vi "daemon.vi"(8 "error in (no error)":errorcluster, 11 "manager_daemon.lvclass":refnum<class "manager_daemon.lvclass">) -> ()   [LabVIEW 2024, in "manager_daemon.lvclass"]
uses:
  manager_daemon.lvclass
  type_defs/cmd--enum.ctl
  TypeDefs/graphic.filter--cluster.ctl
  Graphic_UI/typedefs/volume.type.colors--cluster.ctl
  manager_daemon.lvclass/manager_daemon.ctl
  CV_Shared_Library/volume.type--enum.ctl
  type_defs/msg--cluster.ctl
  type_defs/PublisherData--cluster.ctl
  type_defs/PublisherMap--map.ctl
  add.sub.to.map.vi
  CV_Shared_Library/open.local.volume.file.vi
  add.publisher.vi
  <userlib>/_OpenG.lib/file/file.llb/Strip Path Extension - String__ogtk.vi
  CV_Shared_Library/open.local.issue.file.vi
  CV_Shared_Library/CV_Shared_Library.lvlib
  <userlib>/_OpenG.lib/file/file.llb/openg_file.lvlib
panel:
  out "iteration":i32
  out "latest filter":T1
  out "Volume changed":path
  out "Issue changed":path
  out "cmd":T3
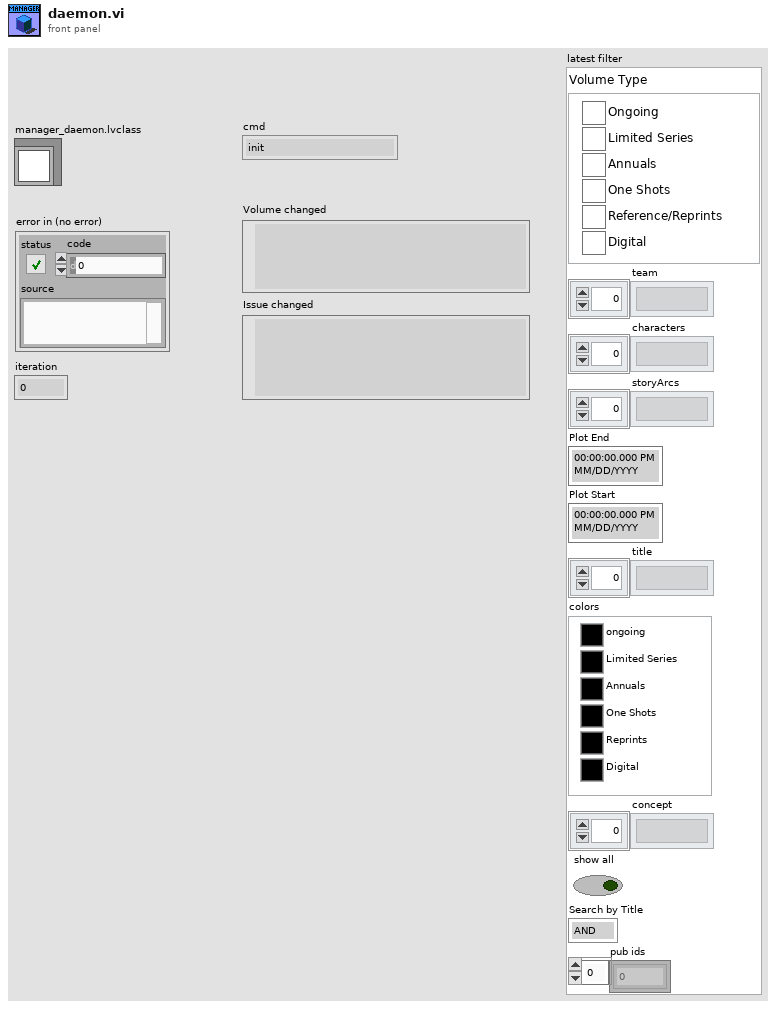
[diagram p1: front panel]
types:
  T1 = typedef "CV_Shared_Library.lvlib/graphic.filter--cluster.ctl" = cluster{"Volume Type":cluster{"Ongoing":bool, "Limited Series":bool, "Annuals":bool, "One Shots":bool, "Reference/Reprints":bool, "Digital":bool}, "team":string[], "characters":string[], "storyArcs":string[], "Plot End":timestamp, "Plot Start":timestamp, "title":string[], "colors":T2, "concept":string[], "show all":bool, "Search by Title":enum32{"AND", "OR"}, "pub ids":i32[]}
  T2 = typedef "volume.type.colors--cluster.ctl" = cluster{"ongoing":u32, "Limited Series":u32, "Annuals":u32, "One Shots":u32, "Reprints":u32, "Digital":u32}
  T3 = typedef "manager_daemon.lvclass/cmd--enum.ctl" = enum16{"init", "run", "load binaries", "save binaries", "updated volume", "get set names", "return vol path by id", "return vol ids by publisher", "display info", "filter release week", "apply filter", "add publisher", "get publishers", "add volume", "save volumes", "add issues", "add issue", "delete volume", "delete issues", "download issues", "scan for reprints", "exit"}
  T4 = cluster{"selection filter":T1, "graph only (f)":bool}
  T5 = cluster{"Volume Path":path, "Update All (T)":bool}
  T6 = typedef "CV_Shared_Library.lvlib/volume.type--enum.ctl" = enum16{"Ongoing", "Limited Series", "Annual", "One Shot", "Reprint/Document", "Digital"}
  T7 = cluster{"search string":string, "source type":T6, "dest type":T6, "publisher":string}
  T8 = typedef "manager_daemon.lvclass/msg--cluster.ctl" = cluster{"cmd":T3, "data":variant}
  T9 = cluster{"Volume Path":i32[], "Update All (T)":bool}
  T10 = cluster{"vol id":i32, "notifier out":refnum<notifier>}
  T11 = cluster{"publisher id":i32, "notifier out":refnum<notifier>}
  T12 = typedef "manager_daemon.lvclass/PublisherData--cluster.ctl" = cluster{"id":i32, "volumes":set{i32}}
  T13 = cluster{"Issue Path":path, "Update All (T)":bool}
  T14 = typedef "manager_daemon.lvclass/sub-map--map.ctl" = map{string, T15}
  T15 = typedef "manager_daemon.lvclass/SubData--cluster.ctl" = cluster{"id":i32, "issues":set{i32}}
  T16 = typedef "manager_daemon.lvclass/binary.references--cluster.ctl" = cluster{"issues.bin ref":refnum<file>, "chars.bin ref":refnum<file>, "concepts.bin ref":refnum<file>, "storys.bin ref":refnum<file>, "teams.bin ref":refnum<file>, "vollumes.bin ref":refnum<file>, "publishers.bin ref":refnum<file>}
  T17 = typedef "manager_daemon.lvclass/VolumeData--cluster.ctl" = cluster{"name":string, "sortable_name":string, "aliases":string[], "description":string, "site_detail_url":string, "count_of_issues":i32, "start_year":i32, "publisher_id":i32, "issue_ids":i32[], "date_last_updated":timestamp, "volume":i32, "cv_id":string, "volume type":T6, "source_path":path}
  T18 = typedef "manager_daemon.lvclass/PublisherMap--map.ctl" = map{string, T12}
  T19 = cluster{"changed volume ids":i32[], "Update All (T)":bool}
  T20 = typedef "CV_RESTful_Lib.lvlib/local_publisher--cluster.ctl" = cluster{"id":i32, "name":string, "sortable_name":string, "aliases":string[], "description":string, "deck":string, "site_detail_url":string, "date_last_updated":timestamp, "cv_id":string, "volume_ids":i32[]}
  T21 = typedef "manager_daemon.lvclass/IssueData--clustrer.ctl" = cluster{"cover_date":timestamp, "cv_id":string, "name":string, "sortable_name":string, "issue_number":string, "deck":string, "description":string, "volume id":i32, "store_date":timestamp, "date_last_updated":timestamp, "site_detail_url":string, "cover_url":string, "source_path":path, "in_collection":bool, "display_date":timestamp}
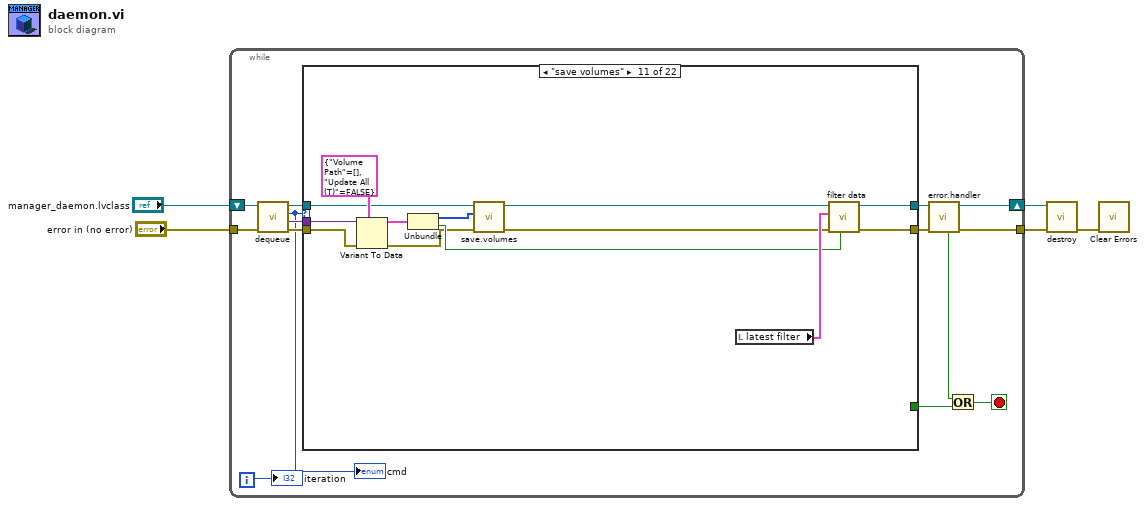
[diagram p0: block diagram]
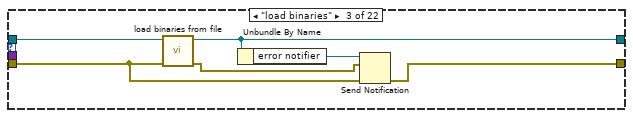
[diagram p4: hidden frame]
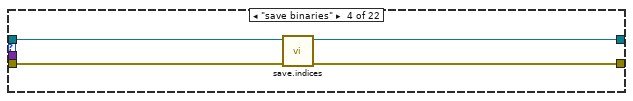
[diagram p5: hidden frame]
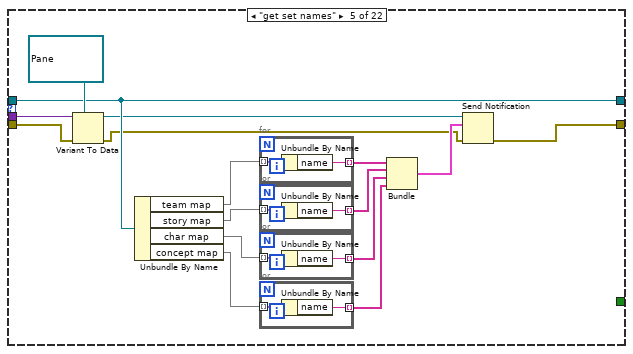
[diagram p6: hidden frame]
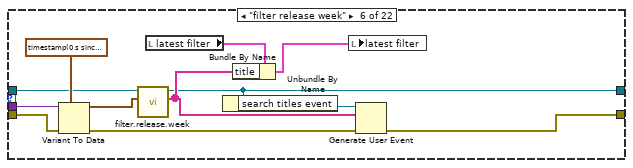
[diagram p7: hidden frame]
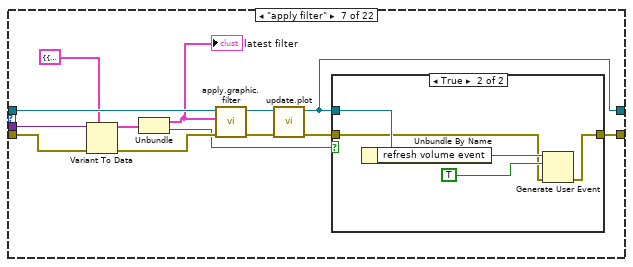
[diagram p8: hidden frame]
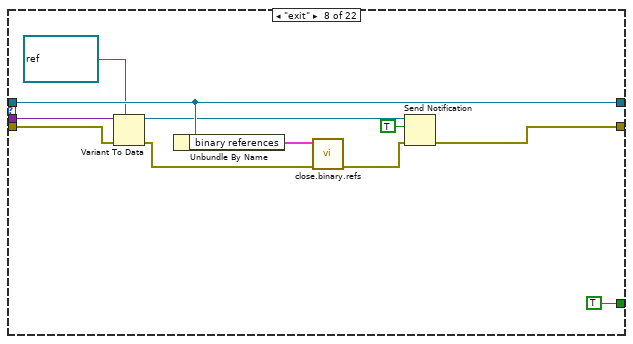
[diagram p10: hidden frame]
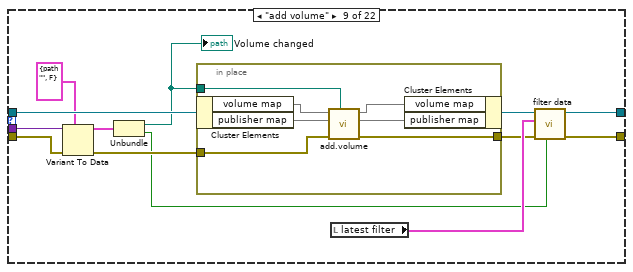
[diagram p11: hidden frame]
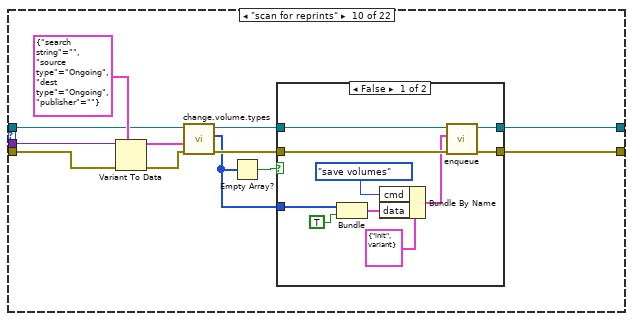
[diagram p12: hidden frame]
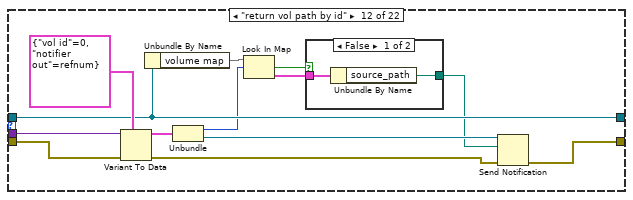
[diagram p14: hidden frame]
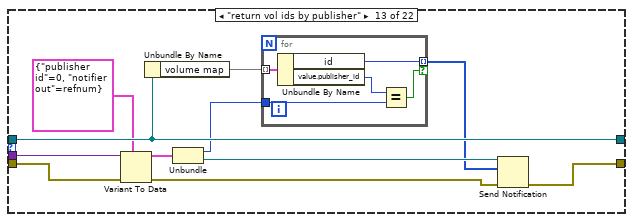
[diagram p16: hidden frame]
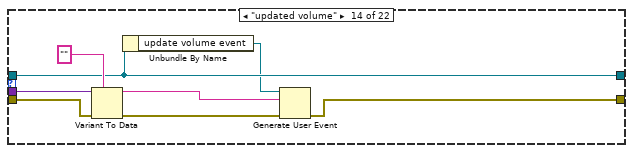
[diagram p17: hidden frame]
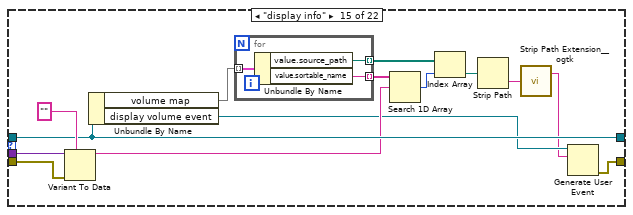
[diagram p18: hidden frame]
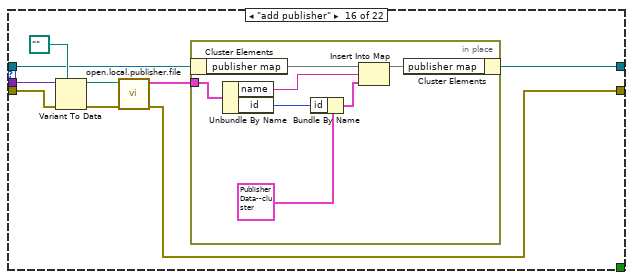
[diagram p19: hidden frame]
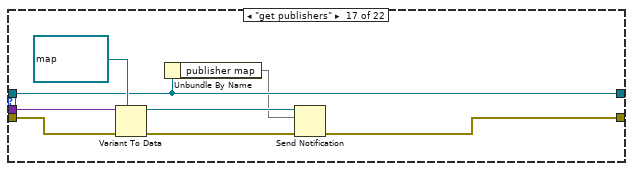
[diagram p20: hidden frame]
diagram:
  n1 = while {
    shift-right: [w11] -> w3
    shift-left: "manager_daemon.lvclass" -> [w19]
    tunnel: "error in (no error)" -> [w18]
    tunnel: [w6] -> w1
    i -> [w13]
    stop <- w8 stop-if-true
    n2 = call "dequeue.vi"("error in (no error)"=w18, "manager_daemon in"=w19) -> ("error out"=w15:errorcluster, "data"=w16:variant, "cmd"=w14:T3, "manager_daemon out"=w17:refnum<class "manager_daemon.lvclass">)  [unwired: 6 in]
    "cmd" <- w14
    n3 = case shown="\"save volumes\"" w14 {
      tunnel: w17 -> [w21 w23 w29 w31 w46 w66 w80 w98 w110 w128 w148 w166 w180 w192 w206 w216 w233 w247 w279 w300 w310 w321]
      tunnel: w16 -> [_ _ _ _ w49 w69 w82 w96 w112 w131 w156 w169 w182 w195 w209 w221 w236 w249 w282 w303 w313 w323]
      tunnel: w15 -> [w20 w22 w26 w33 w47 w67 w81 w94 w111 w130 w155 w168 w181 w193 w208 w220 w235 w248 w281 w302 w312 w322]
      tunnel: [w21 w23 w28 w30 w46 w59 w70 w98 w104 w122 w152 w166 w180 w192 w206 w215 w233 w242 w273 w300 w307 w317] -> w12
      tunnel: [_ _ _ _ _ _ _ TRUE _ _ _ _ _ _ _ _ _ _ _ _ _ _] -> w9
      tunnel: [w20 w22 w24 w32 w34 w60 w75 w89 w105 w121 w153 w159 w176 w188 w198 w213 w229 w245 w274 w296 w304 w315] -> w10
      frame "init" {
      }
      frame "run" {
      }
      frame "load binaries" {
        n4 = call "load binaries from file.vi"("error in (no error)"=w26, "manager_daemon in"=w29) -> ("error out"=w25:errorcluster, "manager_daemon out"=w28:refnum<class "manager_daemon.lvclass">)  [unwired: 8 in]
        n5 = Unbundle By Name(w28) -> ("error notifier"=w27:refnum<notifier>)
        n6 = Send Notification(notification=w25, notifier=w27, error in (no error)=w26) -> (error out=w24:errorcluster)  [unwired: 1 out]
      }
      frame "save binaries" {
        n7 = call "save.indices.vi"("error in (no error)"=w33, "manager_daemon in"=w31) -> ("error out"=w32:errorcluster, "manager_daemon out"=w30:refnum<class "manager_daemon.lvclass">)  [unwired: 8 in]
      }
      frame "get set names" {
        n8 = Variant To Data(error in=w47, type=refnum<notifier> refnum ("notifier out"), Variant=w49) -> (data=w37:refnum<notifier>, error out=w35:errorcluster)
        n9 = Unbundle By Name(w46) -> ("team map"=w45:T14, "story map"=w44:T14, "char map"=w43:T14, "concept map"=w42:T14)
        n10 = for {
          tunnel: w45 -> [w57] mode=indexing
          tunnel: [w56] -> w41 mode=indexing
          n11 = Unbundle By Name(w57) -> ("name"=w56:string)
        }
        n12 = for {
          tunnel: w44 -> [w55] mode=indexing
          tunnel: [w54] -> w40 mode=indexing
          n13 = Unbundle By Name(w55) -> ("name"=w54:string)
        }
        n14 = for {
          tunnel: w43 -> [w53] mode=indexing
          tunnel: [w52] -> w39 mode=indexing
          n15 = Unbundle By Name(w53) -> ("name"=w52:string)
        }
        n16 = for {
          tunnel: w42 -> [w51] mode=indexing
          tunnel: [w50] -> w38 mode=indexing
          n17 = Unbundle By Name(w51) -> ("name"=w50:string)
        }
        n18 = Bundle(w41, w40, w39, w38) -> (w36:cluster{string[], string[], string[], string[]})  [unwired: 1 in]
        n19 = Send Notification(notification=w36, notifier=w37, error in (no error)=w35) -> (error out=w34:errorcluster)  [unwired: 1 out]
      }
      frame "filter release week" {
        n20 = Variant To Data(error in=w67, type=timestamp(0 s since 1904-01-01), Variant=w69) -> (data=w65:timestamp, error out=w61:errorcluster)
        n21 = call "filter.release.week.vi"("date"=w65, "manager_daemon in"=w66) -> ("volume sortable_names"=w62:string[], "manager_daemon out"=w59:refnum<class "manager_daemon.lvclass">)  [unwired: 8 in]
        n22 = local read "latest filter"() -> (w64:T1)
        n23 = Unbundle By Name(w59) -> ("search titles event"=w58:refnum<user-event>)
        n24 = Bundle By Name(cluster=w64, "title"=w62) -> (w63:T1)
        n25 = local write "latest filter"(w63) -> ()
        n26 = Generate User Event(user event=w58, event data cluster=w62, error in=w61) -> (error out=w60:errorcluster)  [unwired: 1 in, 1 out]
      }
      frame "apply filter" {
        n27 = Variant To Data(error in=w81, type=T4 {"selection filter"={"Volume Type"={"Ongoing"=FALSE, "Limited Series"=FALSE, "Annuals"=FALSE, "One Shots"=FALSE, "Reference/Reprints"=FALSE, "Digital"=FALSE}, "team"=[], "characters"=[], "storyArcs"=[], "Plot End"=timestamp(0 s since 1904-01-01), "Plot Start"=timestamp(0 s since 1904-01-01), "title"=[], "colors"={"ongoing"=0, "Limited Series"=0, "Annuals"=0, "One Shots"=0, "Reprints"=0, "Digital"=0}, "concept"=[], "show all"=FALSE, "Search by Title"=enum."AND", "pub ids"=[]}, "graph only (f)"=FALSE} ("output cluster"), Variant=w82) -> (data=w73:T4, error out=w79:errorcluster)
        n28 = Unbundle(w73) -> ("selection filter"=w72:T1, "graph only (f)"=w71:bool)
        "latest filter" <- w72
        n29 = call "apply.graphic.filter.vi"("error in (no error)"=w79, "selection filter"=w72, "manager_daemon in"=w80) -> ("error out"=w77:errorcluster, "manager_daemon out"=w78:refnum<class "manager_daemon.lvclass">)  [unwired: 7 in]
        n30 = call "update.plot.vi"("error in (no error)"=w77, "manager_daemon in"=w78) -> ("error out"=w76:errorcluster, "manager_daemon out"=w70:refnum<class "manager_daemon.lvclass">)  [unwired: 8 in]
        n31 = case shown="True" w71 {
          tunnel: w70 -> [_ w88]
          tunnel: w76 -> [w83 w85]
          tunnel: [w83 w84] -> w75
          frame False {
          }
          frame True {
            n32 = Unbundle By Name(w88) -> ("refresh volume event"=w87:refnum<user-event>)
            n33 = Generate User Event(user event=w87, event data cluster=TRUE ("event data"), error in=w85) -> (error out=w84:errorcluster)  [unwired: 1 in, 1 out]
          }
        }
      }
      frame "exit" {
        n34 = Variant To Data(error in=w94, type=refnum<notifier> refnum ("notifier out"), Variant=w96) -> (data=w92:refnum<notifier>, error out=w93:errorcluster)
        n35 = Unbundle By Name(w98) -> ("binary references"=w97:T16)
        n36 = call "close.binary.refs.vi"("error in"=w93, "binary references"=w97) -> ("error out"=w91:errorcluster)  [unwired: 9 in]
        n37 = Send Notification(notification=TRUE, notifier=w92, error in (no error)=w91) -> (error out=w89:errorcluster)  [unwired: 1 out]
      }
      frame "add volume" {
        n38 = Variant To Data(error in=w111, type=T5 {"Volume Path"=path "", "Update All (T)"=FALSE} ("output cluster"), Variant=w112) -> (data=w102:T5, error out=w109:errorcluster)
        n39 = Unbundle(w102) -> ("Volume Path"=w101:path, "Update All (T)"=w100:bool)
        "Volume changed" <- w101
        n40 = in-place {
          in-place-border: w101 -> [w113]
          in-place-border: w109 -> [w117]
          in-place-border: [w116] -> w106
          n41 = in-place-cluster #1(w110) -> ("volume map"=w119:map{i32, T17}, "publisher map"=w115:T18)
          n42 = call "add.volume.vi"("volume path"=w113, "error in (no error)"=w117, "pub map in"=w115, "volume map in"=w119) -> ("error out"=w116:errorcluster, "pub map out"=w114:T18, "volume map out"=w118:map{i32, T17})  [unwired: 5 in]
          n43 = in-place-cluster #1("volume map"=w118, "publisher map"=w114) -> (w108:refnum<class "manager_daemon.lvclass">)
        }
        n44 = local read "latest filter"() -> (w107:T1)
        n45 = call "filter data.vi"("graph only (f)"=w100, "error in (no error)"=w106, "selection filter"=w107, "manager_daemon in"=w108) -> ("error out"=w105:errorcluster, "manager_daemon out"=w104:refnum<class "manager_daemon.lvclass">)  [unwired: 6 in]
      }
      frame "scan for reprints" {
        n46 = Variant To Data(error in=w130, type=T7 {"search string"="", "source type"=enum."Ongoing", "dest type"=enum."Ongoing", "publisher"=""} ("output cluster"), Variant=w131) -> (data=w126:T7, error out=w127:errorcluster)
        n47 = call "change.volume.types.vi"("error in (no error)"=w127, "change criteria"=w126, "manager_daemon in"=w128) -> ("error out"=w123:errorcluster, "changed volume ids"=w120:i32[], "manager_daemon out"=w124:refnum<class "manager_daemon.lvclass">)  [unwired: 6 in]
        n48 = Empty Array?(array=w120) -> (empty?=w125:bool)
        n49 = case shown="False" w125 {
          tunnel: w124 -> [w141 w143]
          tunnel: w123 -> [w139 w142]
          tunnel: [w140 w143] -> w122
          tunnel: [w138 w142] -> w121
          tunnel: w120 -> [w135 _]
          frame False {
            n50 = Bundle("changed volume ids"=w135, "Update All (T)"=TRUE) -> (w133:T19)  [unwired: 1 in]
            n51 = Bundle By Name(cluster=T8 {"cmd"=enum."init", "data"=variant} ("msg"), "cmd"=cmd--enum."save volumes", "data"=w133) -> (w132:T8)
            n52 = call "enqueue.vi"("error in (no error)"=w139, "msg"=w132, "manager_daemon in"=w141) -> ("error out"=w138:errorcluster, "manager_daemon out"=w140:refnum<class "manager_daemon.lvclass">)  [unwired: 7 in]
          }
          frame True {
          }
        }
      }
      frame "save volumes" {
        n53 = Variant To Data(error in=w155, type=T9 {"Volume Path"=[], "Update All (T)"=FALSE} ("output cluster"), Variant=w156) -> (data=w150:T9, error out=w147:errorcluster)
        n54 = Unbundle(w150) -> ("Volume Path"=w144:i32[], "Update All (T)"=w149:bool)
        n55 = call "save.volumes.vi"("error in (no error)"=w147, "volume ids"=w144, "manager_daemon in"=w148) -> ("error out"=w145:errorcluster, "manager_daemon out"=w146:refnum<class "manager_daemon.lvclass">)  [unwired: 7 in]
        n56 = local read "latest filter"() -> (w154:T1)
        n57 = call "filter data.vi"("graph only (f)"=w149, "error in (no error)"=w145, "selection filter"=w154, "manager_daemon in"=w146) -> ("error out"=w153:errorcluster, "manager_daemon out"=w152:refnum<class "manager_daemon.lvclass">)  [unwired: 6 in]
      }
      frame "return vol path by id" {
        n58 = Variant To Data(error in=w168, type=T10 {"vol id"=0, "notifier out"=refnum} ("output cluster"), Variant=w169) -> (data=w164:T10, error out=w160:errorcluster)
        n59 = Unbundle By Name(w166) -> ("volume map"=w165:map{i32, T17})
        n60 = Unbundle(w164) -> ("vol id"=w163:i32, "notifier out"=w161:refnum<notifier>)
        n61 = Look In Map(map=w165, key=w163) -> (key not found?=w157:bool, value=w162:T17)  [unwired: 1 in]
        n62 = case shown="False" w157 {
          tunnel: w162 -> [w171 _]
          tunnel: [w170 _] -> w158
          frame False {
            n63 = Unbundle By Name(w171) -> ("source_path"=w170:path)
          }
          frame True {
          }
        }
        n64 = Send Notification(notification=w158, notifier=w161, error in (no error)=w160) -> (error out=w159:errorcluster)  [unwired: 1 out]
      }
      frame "return vol ids by publisher" {
        n65 = Variant To Data(error in=w181, type=T11 {"publisher id"=0, "notifier out"=refnum} ("output cluster"), Variant=w182) -> (data=w179:T11, error out=w177:errorcluster)
        n66 = Unbundle By Name(w180) -> ("volume map"=w174:map{i32, T17})
        n67 = Unbundle(w179) -> ("publisher id"=w173:i32, "notifier out"=w178:refnum<notifier>)
        n68 = for {
          tunnel: w174 -> [w187] mode=indexing
          tunnel: w173 -> [w185]
          tunnel: [w184] -> w172 mode=indexing if=w183
          n69 = Unbundle By Name(w187) -> ("id"=w184:i32, "value.publisher_id"=w186:i32)
          n70 = Equal?(x=w186, y=w185) -> (x = y?=w183:bool)
        }
        n71 = Send Notification(notification=w172, notifier=w178, error in (no error)=w177) -> (error out=w176:errorcluster)  [unwired: 1 out]
      }
      frame "updated volume" {
        n72 = Variant To Data(error in=w193, type="", Variant=w195) -> (data=w191:string, error out=w190:errorcluster)
        n73 = Unbundle By Name(w192) -> ("update volume event"=w189:refnum<user-event>)
        n74 = Generate User Event(user event=w189, event data cluster=w191, error in=w190) -> (error out=w188:errorcluster)  [unwired: 1 in, 1 out]
      }
      frame "display info" {
        n75 = Variant To Data(error in=w208, type="", Variant=w209) -> (data=w203:string)  [unwired: 1 out]
        n76 = Unbundle By Name(w206) -> ("volume map"=w205:map{i32, T17}, "display volume event"=w197:refnum<user-event>)
        n77 = for {
          tunnel: w205 -> [w212] mode=indexing
          tunnel: [w211] -> w204 mode=indexing
          tunnel: [w210] -> w201 mode=indexing
          n78 = Unbundle By Name(w212) -> ("value.source_path"=w210:path, "value.sortable_name"=w211:string)
        }
        n79 = Search 1D Array(1D array=w204, element=w203) -> (index of element=w202:i32)  [unwired: 1 in]
        n80 = Index Array(array=w201, index=w202) -> (element=w200:path)
        n81 = Strip Path(path=w200) -> (name=w199:string)  [unwired: 1 out]
        n82 = call-poly <userlib>:"Strip Path Extension__ogtk.vi"("path"=w199) -> ("root"=w196:string)  [unwired: 1 out]
        n83 = Generate User Event(user event=w197, event data cluster=w196) -> (error out=w198:errorcluster)  [unwired: 2 in, 1 out]
      }
      frame "add publisher" {
        n84 = Variant To Data(error in=w220, type=path "", Variant=w221) -> (data=w218:path, error out=w217:errorcluster)
        n85 = call "open.local.publisher.file.vi"("error in (no error)"=w217, "publisher json"=w218) -> ("error out"=w213:errorcluster, "publisher"=w214:T20)  [unwired: 8 in]
        n86 = in-place {
          in-place-border: w214 -> [w226]
          n87 = in-place-cluster #2(w216) -> ("publisher map"=w228:T18)
          n88 = Unbundle By Name(w226) -> ("name"=w225:string, "id"=w224:i32)
          n89 = Bundle By Name(cluster=T12 {"id"=0, "volumes"={}} ("value"), "id"=w224) -> (w222:T12)
          n90 = Insert Into Map(map in=w228, key=w225, value=w222) -> (map out=w227:T18)  [unwired: 2 out]
          n91 = in-place-cluster #2("publisher map"=w227) -> (w215:refnum<class "manager_daemon.lvclass">)
        }
      }
      frame "get publishers" {
        n92 = Variant To Data(error in=w235, type=refnum<notifier> refnum ("notifier out"), Variant=w236) -> (data=w232:refnum<notifier>, error out=w231:errorcluster)
        n93 = Unbundle By Name(w233) -> ("publisher map"=w230:T18)
        n94 = Send Notification(notification=w230, notifier=w232, error in (no error)=w231) -> (error out=w229:errorcluster)  [unwired: 1 out]
      }
      frame "add issue" {
        n95 = Variant To Data(error in=w248, type=T13 {"Issue Path"=path "", "Update All (T)"=FALSE} ("output cluster"), Variant=w249) -> (data=w240:T13, error out=w246:errorcluster)
        n96 = Unbundle(w240) -> ("Issue Path"=w239:path, "Update All (T)"=w238:bool)
        "Issue changed" <- w239
        n97 = in-place {
          in-place-border: w239 -> [w270]
          in-place-border: w246 -> [w259]
          in-place-border: [w258] -> w243
          n98 = in-place-cluster #3(w247) -> ("issue map"=w269:map{i32, T21}, "char map"=w267:T14, "concept map"=w265:T14, "story map"=w263:T14, "team map"=w261:T14)
          n99 = call "add.issue.vi"("issues in"=w269, "Path"=w270, "char map in"=w267, "concept map in"=w265, "story map in"=w263, "error in (no error)"=w259, "team map in"=w261) -> ("issues out"=w268:map{i32, T21}, "char map out"=w266:T14, "concept map out"=w264:T14, "story map out"=w262:T14, "team map out"=w260:T14, "error out"=w258:errorcluster)  [unwired: 3 in]
          n100 = in-place-cluster #3("issue map"=w268, "char map"=w266, "concept map"=w264, "story map"=w262, "team map"=w260) -> (w244:refnum<class "manager_daemon.lvclass">)
        }
        n101 = local read "latest filter"() -> (w237:T1)
        n102 = case shown="True" w238 {
          tunnel: w237 -> [_ w252]
          tunnel: [w250 w254] -> w245
          tunnel: w244 -> [w251 w257]
          tunnel: w243 -> [w250 w256]
          tunnel: [w251 w255] -> w242
          frame False {
          }
          frame True {
            n103 = call "filter data.vi"("graph only (f)"=FALSE, "error in (no error)"=w256, "selection filter"=w252, "manager_daemon in"=w257) -> ("error out"=w254:errorcluster, "manager_daemon out"=w255:refnum<class "manager_daemon.lvclass">)  [unwired: 6 in]
          }
        }
      }
      frame "add issues" {
        n104 = Variant To Data(error in=w281, type=path[] [], Variant=w282) -> (data=w277:path[], error out=w278:errorcluster)
        n105 = in-place {
          in-place-border: w277 -> [w295]
          in-place-border: w278 -> [w284]
          in-place-border: [w283] -> w275
          n106 = in-place-cluster #4(w279) -> ("issue map"=w294:map{i32, T21}, "char map"=w292:T14, "concept map"=w290:T14, "story map"=w288:T14, "team map"=w286:T14)
          n107 = call "add.issues.vi"("issues in"=w294, "Array"=w295, "char map in"=w292, "concept map in"=w290, "story map in"=w288, "error in (no error)"=w284, "team map in"=w286) -> ("issues out"=w293:map{i32, T21}, "char map out"=w291:T14, "concept map out"=w289:T14, "story map out"=w287:T14, "team map out"=w285:T14, "error out"=w283:errorcluster)  [unwired: 3 in]
          n108 = in-place-cluster #4("issue map"=w293, "char map"=w291, "concept map"=w289, "story map"=w287, "team map"=w285) -> (w276:refnum<class "manager_daemon.lvclass">)
        }
        n109 = local read "latest filter"() -> (w272:T1)
        n110 = call "filter data.vi"("graph only (f)"=FALSE, "error in (no error)"=w275, "selection filter"=w272, "manager_daemon in"=w276) -> ("error out"=w274:errorcluster, "manager_daemon out"=w273:refnum<class "manager_daemon.lvclass">)  [unwired: 6 in]
      }
      frame "download issues" {
        n111 = Variant To Data(error in=w302, type=i32[] [], Variant=w303) -> (data=w298:i32[], error out=w297:errorcluster)
        n112 = Unbundle By Name(w300) -> ("download issues event"=w299:refnum<user-event>)
        n113 = Generate User Event(user event=w299, event data cluster=w298, error in=w297) -> (error out=w296:errorcluster)  [unwired: 1 in, 1 out]
      }
      frame "delete volume" {
        n114 = Variant To Data(error in=w312, type=path "", Variant=w313) -> (data=w309:path, error out=w306:errorcluster)
        n115 = call "remove.volume.vi"("Path"=w309, "manager_daemon in"=w310) -> ("manager_daemon out"=w308:refnum<class "manager_daemon.lvclass">)  [unwired: 9 in]
        n116 = local write "Volume changed"(w309) -> ()
        n117 = local read "latest filter"() -> (w305:T1)
        n118 = call "filter data.vi"("error in (no error)"=w306, "selection filter"=w305, "manager_daemon in"=w308) -> ("error out"=w304:errorcluster, "manager_daemon out"=w307:refnum<class "manager_daemon.lvclass">)  [unwired: 7 in]
      }
      frame "delete issues" {
        n119 = Variant To Data(error in=w322, type=path[] [], Variant=w323) -> (data=w319:path[], error out=w316:errorcluster)
        n120 = call "remove.issue.vi"("issue path"=w319, "manager_daemon in"=w321) -> ("manager_daemon out"=w318:refnum<class "manager_daemon.lvclass">)  [unwired: 9 in]
        n121 = local read "latest filter"() -> (w314:T1)
        n122 = call "filter data.vi"("error in (no error)"=w316, "selection filter"=w314, "manager_daemon in"=w318) -> ("error out"=w315:errorcluster, "manager_daemon out"=w317:refnum<class "manager_daemon.lvclass">)  [unwired: 7 in]
      }
    }
    n123 = call "error.handler.vi"("error in (no error)"=w10, "manager_daemon in"=w12) -> ("error out"=w6:errorcluster, "manager_daemon out"=w11:refnum<class "manager_daemon.lvclass">, "exit"=w7:bool)  [unwired: 7 in]
    n124 = Or(x=w7, y=w9) -> (x .or. y?=w8:bool)
    "iteration" <- w13
  }
  n125 = call "destroy.vi"("error in (no error)"=w1, "manager_daemon in"=w3) -> ("error out"=w2:errorcluster)  [unwired: 8 in, 1 out]
  n126 = call <vilib>:"Clear Errors.vi"("error in (no error)"=w2) -> ()  [unwired: 5 in, 2 out]
